vi "ParsingSpreadString.vi"(10 "구분 문자":string, 11 "문자열":string) -> (3 "result":string[](array[string]))   [LabVIEW 2018, in "Library-DataConvert.lvlib"]
uses:
  Library-DataConvert.lvlib
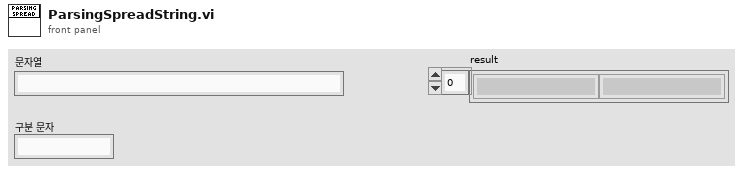
[diagram p1: front panel]
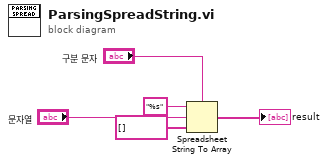
[diagram p0: block diagram]
diagram:
  n1 = Spreadsheet String To Array(delimiter (Tab)="구분 문자", format string="%s", spreadsheet string="문자열", array type (2D Dbl)=string[] []) -> (array=→"result":string[])
